vi "Launch Executable w-Command Line Parameters.vi"(4 "Error In":errorcluster, 6 "Command Line Parameters":string, 7 "Path to Executable":path) -> (0 "Error Out":errorcluster)   [LabVIEW 2014, in "Managing Executables.lvlib"]
uses:
  Managing Executables.lvlib
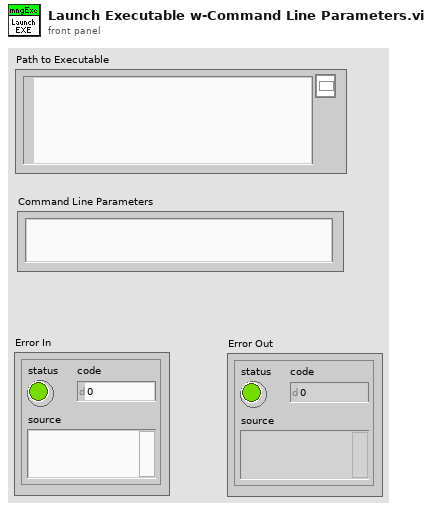
[diagram p1: front panel]
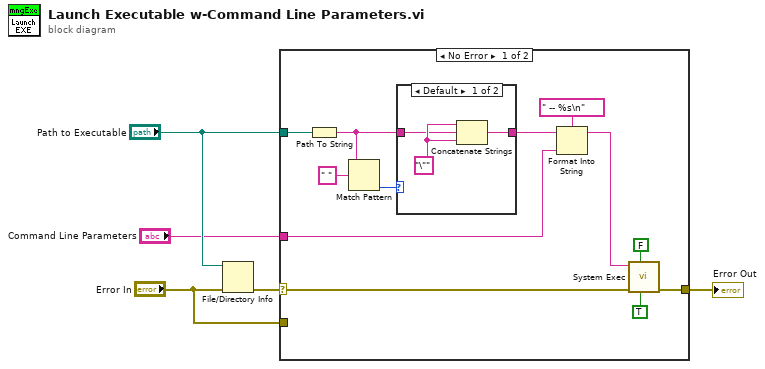
[diagram p0: block diagram]
diagram:
  n1 = File/Directory Info(path="Path to Executable", error in="Error In") -> (error out=w3:errorcluster)  [unwired: 6 out]
  n2 = case shown="No Error" w3 {
    selector: w3 -> [w7 _]
    tunnel: [w6 w22] -> w5
    tunnel: "Path to Executable" -> [w12 _]
    tunnel: "Error In" -> [_ w22]
    tunnel: "Command Line Parameters" -> [w9 _]
    frame No Error {
      n3 = Path To String(path=w12) -> (string=w13:string)
      n4 = Match Pattern(string=w13, regular expression=" ") -> (offset past match=w14:i32)  [unwired: 1 in, 3 out]
      n5 = case shown="Default" w14 {
        tunnel: w13 -> [w18 w21]
        tunnel: [w20 w21] -> w10
        frame Default {
          w19 = "\"" ("regular expression")
          n6 = Concatenate Strings(w19, w18, w19) -> (w20:string)
        }
        frame -1 {
        }
      }
      n7 = Format Into String(format string=" -- %s\n", initial string=w10, w9) -> (resulting string=w8:string)  [unwired: 1 in, 1 out]
      n8 = call <vilib>:"System Exec.vi"("run minimized? (F)"=TRUE, "wait until completion? (T)"=FALSE, "error in (no error)"=w7, "command line"=w8) -> ("error out"=w6:errorcluster)  [unwired: 4 in, 3 out]
    }
    frame Error {
    }
  }
  "Error Out" <- w5
